vi "Discover Plugins.vi"(8 "error in (no error)":errorcluster, 11 "CIFPluginManager in":refnum<class "CIFPluginManager.lvclass">) -> (0 "error out":errorcluster, 3 "CIFPluginManager out":refnum<class "CIFPluginManager.lvclass">)   [LabVIEW 2021, in "CIFPluginManager.lvclass"]
uses:
  CIFPluginManager.lvclass
  typedef/Discovered Plugin.ctl
  CIFCore/Common/Typedef/Version.ctl
  <vilib>/Utility/miscctls.llb/LVMapReplaceAction.ctl
  CIFPluginManager.lvclass/CIFPluginManager.ctl
  CIFCore/Common/CIFCoreCommon.lvlib
  typedef/Plugin Metadata.ctl
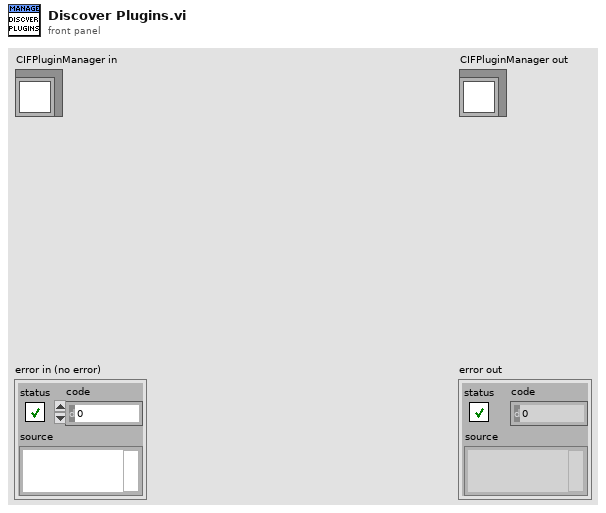
[diagram p1: front panel]
types:
  T1 = typedef "CIFPluginManager.lvclass/Discovered Plugin.ctl" = cluster{"Filename":string, "Plugin Type":string, "Qualified name":string, "Version":T2, "Plugin Metadata":T3}
  T2 = typedef "CIFCoreCommon.lvlib/Version.ctl" = cluster{"Major":i32, "Minor":i32, "Fix":i32, "Build":i32}
  T3 = typedef "CIFPluginManager.lvclass/Plugin Metadata.ctl" = cluster{"Description":string, "History":string, "Author":string}
  T4 = typedef "LVMapReplaceAction.ctl" = enum32{"Modify Entry only if found", "Add or Modify Entry", "Delete Entry"}
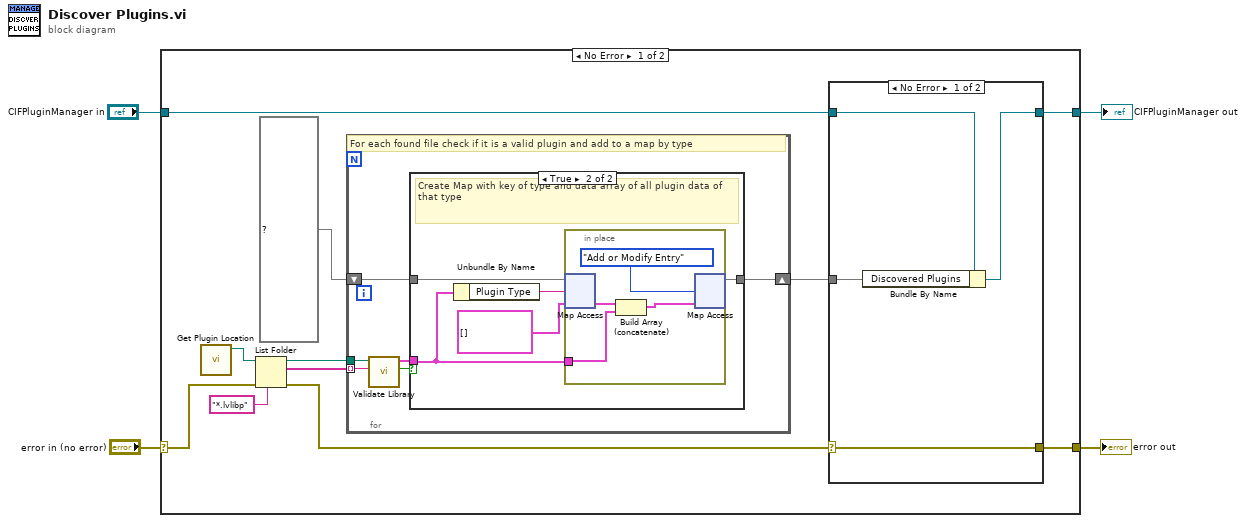
[diagram p0: block diagram]
diagram:
  n1 = case shown="No Error" "error in (no error)" {
    selector: "error in (no error)" -> [w13 w39]
    tunnel: [w8 w39] -> w3
    tunnel: [w7 w38] -> w1
    tunnel: "CIFPluginManager in" -> [w10 w38]
    frame No Error {
      n2 = call "Get Plugin Location.vi"() -> ("Plugin Directory"=w12:path)  [unwired: 11 in]
      n3 = List Folder(path=w12, pattern="*.lvlibp", error in=w13) -> (path out=w14:path, filenames=w15:string[], error out=w9:errorcluster)  [unwired: 1 in, 1 out]
      n4 = for {
        tunnel: w15 -> [w26] mode=indexing
        tunnel: w14 -> [w27]
        shift-right: [w22] -> w6
        shift-left: map{string, T1[]} {} ("map") -> [w24]
        # "For each found file check if it is a valid plugin and add to a map by type"
        n5 = call "Validate Library.vi"("Filename"=w26, "path in"=w27) -> ("valid"=w25:bool, "Discovered Plugin"=w23:T1)  [unwired: 8 in]
        n6 = case shown="True" w25 {
          tunnel: w24 -> [w28 w33]
          tunnel: w23 -> [_ w30]
          tunnel: [w28 w29] -> w22
          frame False {
          }
          frame True {
            # "Create Map with key of type and data array of all plugin data of that type"
            n7 = Unbundle By Name(w30) -> ("Plugin Type"=w32:string)
            n8 = in-place {
              in-place-border: w30 -> [w35]
              n9 = in-place-map #1(w33, w32, T1[] [] ("value")) -> (w36:T1[])  [unwired: 1 out]
              n10 = Build Array (concatenate)(w36, w35) -> (w34:T1[])
              n11 = in-place-map #1(w34, LVMapReplaceAction."Add or Modify Entry" ("action")) -> (w29:map{string, T1[]})  [unwired: 2 out]
            }
          }
        }
      }
      n12 = case shown="No Error" w9 {
        selector: w9 -> [w19 w20]
        tunnel: w10 -> [w18 w21]
        tunnel: [w19 w20] -> w8
        tunnel: w6 -> [w17 _]
        tunnel: [w16 w21] -> w7
        frame No Error {
          n13 = Bundle By Name(cluster=w18, "Discovered Plugins"=w17) -> (w16:refnum<class "CIFPluginManager.lvclass">)
        }
        frame Error {
        }
      }
    }
    frame Error {
    }
  }
  "error out" <- w3
  "CIFPluginManager out" <- w1
